vi "Add File to Project Item.vi"(8 "error in":errorcluster, 10 "File Paths":path[](array[path]), 11 "Item ref in":refnum<vi>) -> (0 "error out":errorcluster, 3 "Item ref out":refnum<vi>)   [LabVIEW 2019, in "Project Sync Tools.lvclass"]
uses:
  Project Sync Tools.lvclass
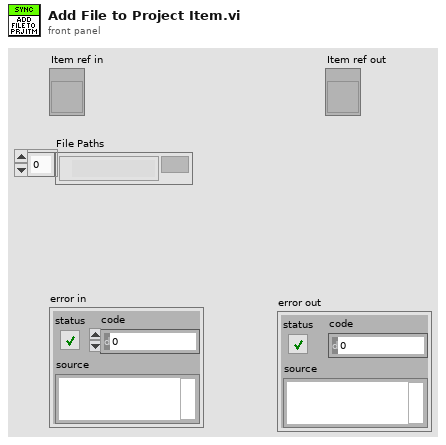
[diagram p1: front panel]
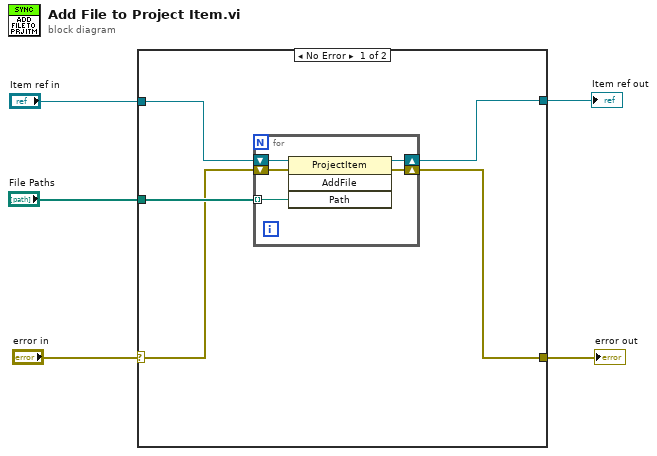
[diagram p0: block diagram]
diagram:
  n1 = case shown="No Error" "error in" {
    selector: "error in" -> [w8 w17]
    tunnel: "File Paths" -> [w10 _]
    tunnel: "Item ref in" -> [w9 w16]
    tunnel: [w7 w17] -> w3
    tunnel: [w6 w16] -> w1
    frame No Error {
      n2 = for {
        shift-right: [w13] -> w7
        shift-left: w8 -> [w15]
        tunnel: w10 -> [w12] mode=indexing
        shift-right: [w11] -> w6
        shift-left: w9 -> [w14]
        n3 = invoke class="ProjectItem" method="AddFile"(reference=w14, error in=w15, "Path"=w12) -> (reference out=w11:refnum<vi>, error out=w13:errorcluster)  [unwired: 1 in, 2 out]
      }
    }
    frame Error {
    }
  }
  "error out" <- w3
  "Item ref out" <- w1
